vi "Toggle Control 9620.vi"(8 "error in (no error)":errorcluster, 11 "VISA resource name":refnum<visa-resource-name>="COM3") -> (0 "error out":errorcluster, 3 "VISA resource name out":refnum<visa-resource-name>)   [LabVIEW 2023]
doc: "This changes the temperature setpoint. If you want to query the setpoint after this, make sure there is a 0.2 s delay (according to manual)."
panel:
  out "Command string":string="S"
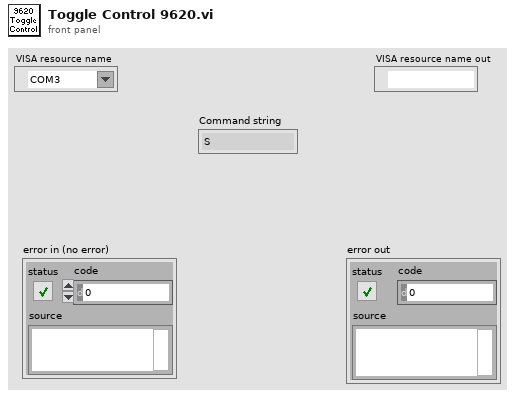
[diagram p1: front panel]
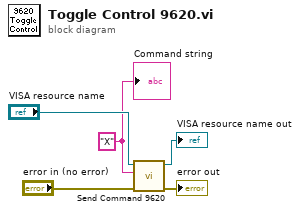
[diagram p0: block diagram]
diagram:
  w1 = "X"
  n1 = call "Send Command 9620.vi"("error in (no error)"="error in (no error)", "command"=w1, "VISA resource name"="VISA resource name") -> ("error out"=→"error out":errorcluster, "VISA resource name out"=→"VISA resource name out":refnum<visa-resource-name>)  [unwired: 7 in]
  "Command string" <- w1
